vi "ReceiveADCdata.vi"(8 "error in (no error)":errorcluster, 11 "Model Driver in":refnum<class "Model Driver.lvclass">) -> (0 "error out":errorcluster, 3 "Model Driver out":refnum<class "Model Driver.lvclass">)   [LabVIEW 2023, in "Model Driver.lvclass"]
doc: "Receives the Single Channel digital data and multichannel digital data in an U8 array from the ADC conversion class."
uses:
  Model Driver.lvclass
  Conversion/Conversion.lvclass
  Model Driver.lvclass/Model Driver.ctl
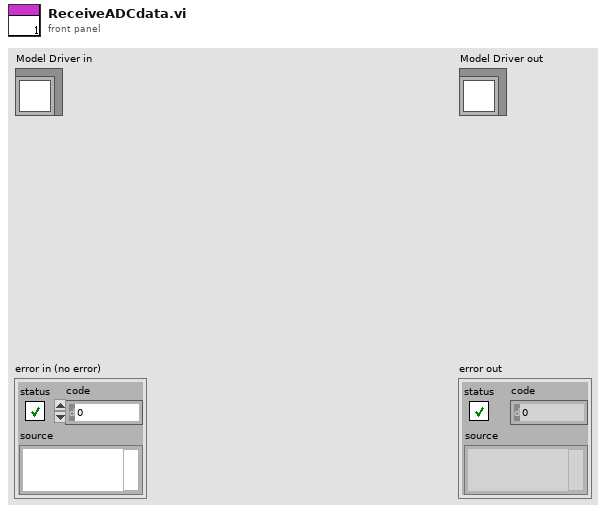
[diagram p1: front panel]
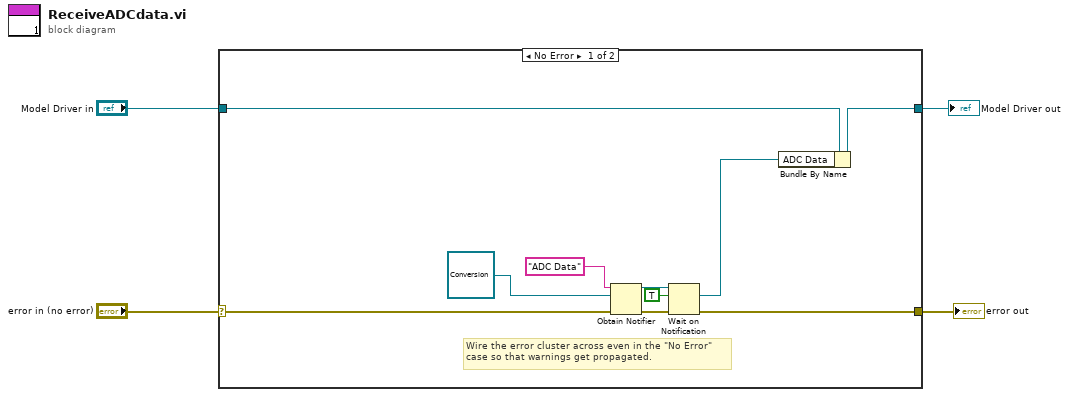
[diagram p0: block diagram]
diagram:
  n1 = case shown="No Error" "error in (no error)" {
    selector: "error in (no error)" -> [w9 w16]
    tunnel: [w8 w16] -> w3
    tunnel: [w7 w15] -> w1
    tunnel: "Model Driver in" -> [w14 w15]
    frame No Error {
      # "Wire the error cluster across even in the \"No Error\"\ncase so that warnings get propagated."
      n2 = Obtain Notifier(name (unnamed)="ADC Data", notification data type=refnum<class "Conversion.lvclass"> refnum ("ADC Class .Selected Channel"), error in (no error)=w9) -> (notifier out=w12:refnum<notifier>, error out=w13:errorcluster)  [unwired: 1 in, 1 out]
      n3 = Wait on Notification(notifier=w12, ignore previous (F)=TRUE, error in (no error)=w13) -> (notification=w5:refnum<class "Conversion.lvclass">, error out=w8:errorcluster)  [unwired: 1 in, 2 out]
      n4 = Bundle By Name(cluster=w14, "ADC Data"=w5) -> (w7:refnum<class "Model Driver.lvclass">)
    }
    frame Error {
    }
  }
  "error out" <- w3
  "Model Driver out" <- w1
